vi "mdps_global.vi"() -> ()   [LabVIEW 2015]
panel:
  in  "Duty Cycle":dbl(knob)=0.05 min=0.05 max=0.1 step=0.001 scale=0.05..0.1
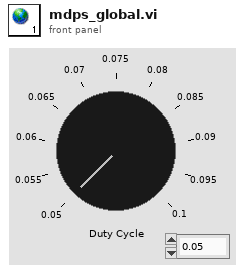
[diagram p1: front panel]
diagram:
